vi "GetBarHeight.vi"(8 "error in (no error)":errorcluster, 11 "EAN-13 in":refnum<class "EAN-13.lvclass">) -> (0 "error out":errorcluster, 2 "Bar Height":u8=76, 3 "EAN-13 out":refnum<class "EAN-13.lvclass">)   [LabVIEW 2013, in "BarCodes.lvlib" / "EAN-13.lvclass"]
uses:
  EAN-13.lvclass
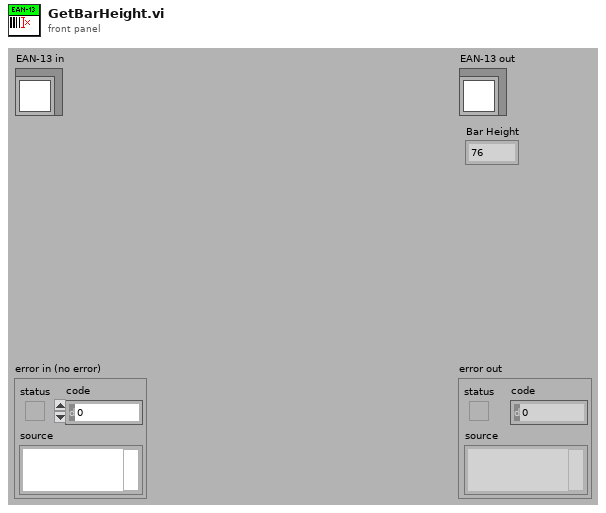
[diagram p1: front panel]
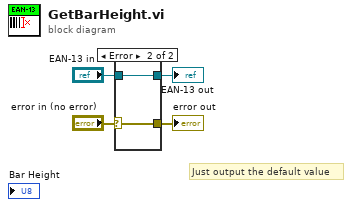
[diagram p0: block diagram]
diagram:
  # "Just output the default value"
  n1 = case shown="Error" "error in (no error)" {
    selector: "error in (no error)" -> [w6 w7]
    tunnel: [w6 w7] -> w3
    tunnel: "EAN-13 in" -> [w5 w8]
    tunnel: [w5 w8] -> w1
    frame No Error {
    }
    frame Error {
    }
  }
  "error out" <- w3
  "EAN-13 out" <- w1
